vi "开机界面.vi"   [LabVIEW 2011]
types:
  T1 = enum32{"Invalid", "Standard", "Closed", "Hidden", "Minimized", "Maximized"}
  T2 = enum16{"Always On", "Always Off", "Off While Running"}
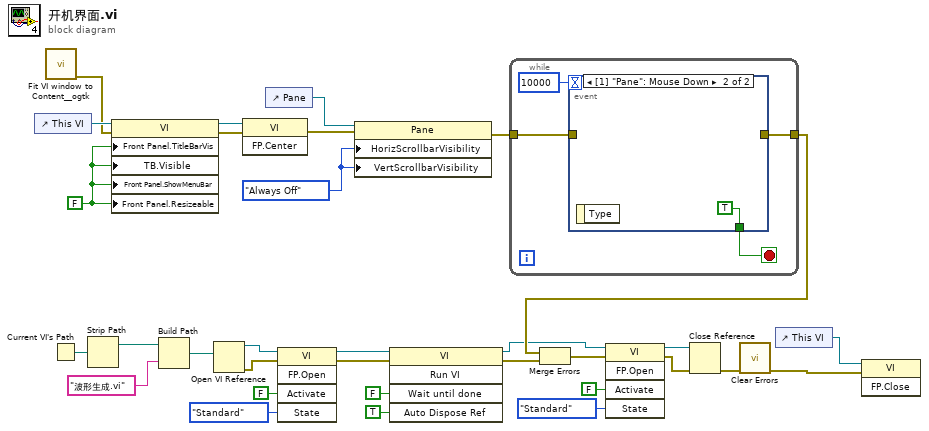
[diagram p0: block diagram]
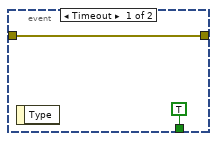
[diagram p2: hidden frame]
diagram:
  w25 = FALSE ("Front Panel Window:Resizable")
  w26 = T2."Always Off" ("Vertical Scrollbar Visibility")
  n1 = control-ref of="This VI"() -> (w32:refnum<vi>)
  n2 = call <userlib>:"Fit VI window to Content__ogtk.vi"() -> ("error out"=w31:errorcluster)  [unwired: 6 in, 1 out]
  n3 = Current VI's Path() -> (path=w23:path)
  n4 = Strip Path(path=w23) -> (stripped path=w22:path)  [unwired: 1 out]
  n5 = property class="VI"(reference=w32, error in=w31, "Front Panel.TitleBarVis"=w25, "TB.Visible"=w25, "Front Panel.ShowMenuBar"=w25, "Front Panel.Resizeable"=w25) -> (reference out=w30:refnum<vi>, error out=w29:errorcluster)
  n6 = Build Path(base path=w22, name or relative path="波形生成.vi") -> (appended path=w21:path)
  n7 = Open VI Reference(vi path=w21) -> (vi reference=w19:refnum<vi>, error out=w18:errorcluster)  [unwired: 5 in]
  n8 = invoke class="VI" method="FP.Center"(reference=w30, error in=w29) -> (error out=w28:errorcluster)  [unwired: 1 in, 2 out]
  n9 = control-ref of="Pane"() -> (w27:refnum<vi>)
  n10 = invoke class="VI" method="FP.Open"(reference=w19, error in=w18, "Activate"=FALSE ("Activate?"), "State"=T1."Standard") -> (reference out=w15:refnum<vi>, error out=w14:errorcluster)  [unwired: 1 in, 3 out]
  n11 = property class="Pane"(reference=w27, error in=w28, "HorizScrollbarVisibility"=w26, "VertScrollbarVisibility"=w26) -> (error out=w24:errorcluster)  [unwired: 1 out]
  n12 = invoke class="VI" method="Run VI"(reference=w15, error in=w14, "Wait until done"=FALSE ("Wait Until Done"), "Auto Dispose Ref"=TRUE ("Auto Dispose Reference")) -> (reference out=w8:refnum<vi>, error out=w11:errorcluster)  [unwired: 1 in, 3 out]
  n13 = while {
    tunnel: w24 -> [w36]
    tunnel: [w35] -> w10
    stop <- w33 stop-if-true
    n14 = event shown="[1] \"Pane\": Mouse Down" {
      selector: _ -> [_ _]
      dyn-events: _ -> [_ _]
      timeout: 10000 -> [_ _]
      tunnel: [w38 _] -> w35
      tunnel: w36 -> [w38 _]
      tunnel: [TRUE TRUE] -> w33
      event Timeout {
        n15 = event-data() -> ()  [unwired: 1 in, 1 out]
      }
      event Mouse Down {
        n16 = event-data() -> ()  [unwired: 1 in, 1 out]
      }
    }
  }
  n17 = Merge Errors(w10, w11) -> (w9:errorcluster)
  n18 = invoke class="VI" method="FP.Open"(reference=w8, error in=w9, "Activate"=FALSE ("Activate?"), "State"=T1."Standard") -> (reference out=w5:refnum<vi>, error out=w4:errorcluster)  [unwired: 1 in, 3 out]
  n19 = Close Reference(reference=w5, error in (no error)=w4) -> (error out=w3:errorcluster)
  n20 = call <vilib>:"Clear Errors.vi"("error in (no error)"=w3) -> ("error out"=w2:errorcluster)  [unwired: 6 in]
  n21 = control-ref of="This VI"() -> (w1:refnum<vi>)
  n22 = invoke class="VI" method="FP.Close"(reference=w1, error in=w2) -> ()  [unwired: 1 in, 3 out]
